vi "Update Accessory Info Tree.vi"(8 "error in":errorcluster, 9 "Devs with Inserted/Removed Accessories":string[](array[string]), 10 "All Devices":tag[](array[tag]), 11 "Accessory Info Tree":refnum<vi>) -> (0 "error out":errorcluster)   [LabVIEW 2022 SP3]
doc: "This VI updates a tree control to display DAQmx device and accessory information."
uses:
  <resource>/objmgr/daqmx.rc
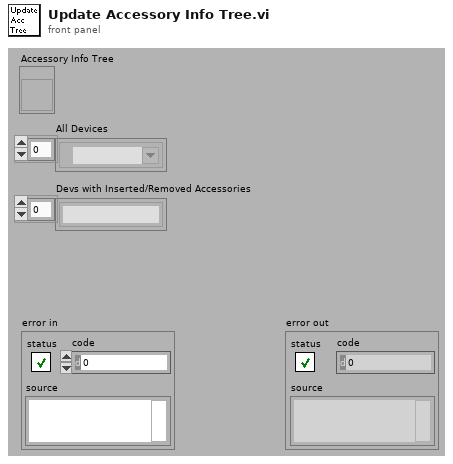
[diagram p1: front panel]
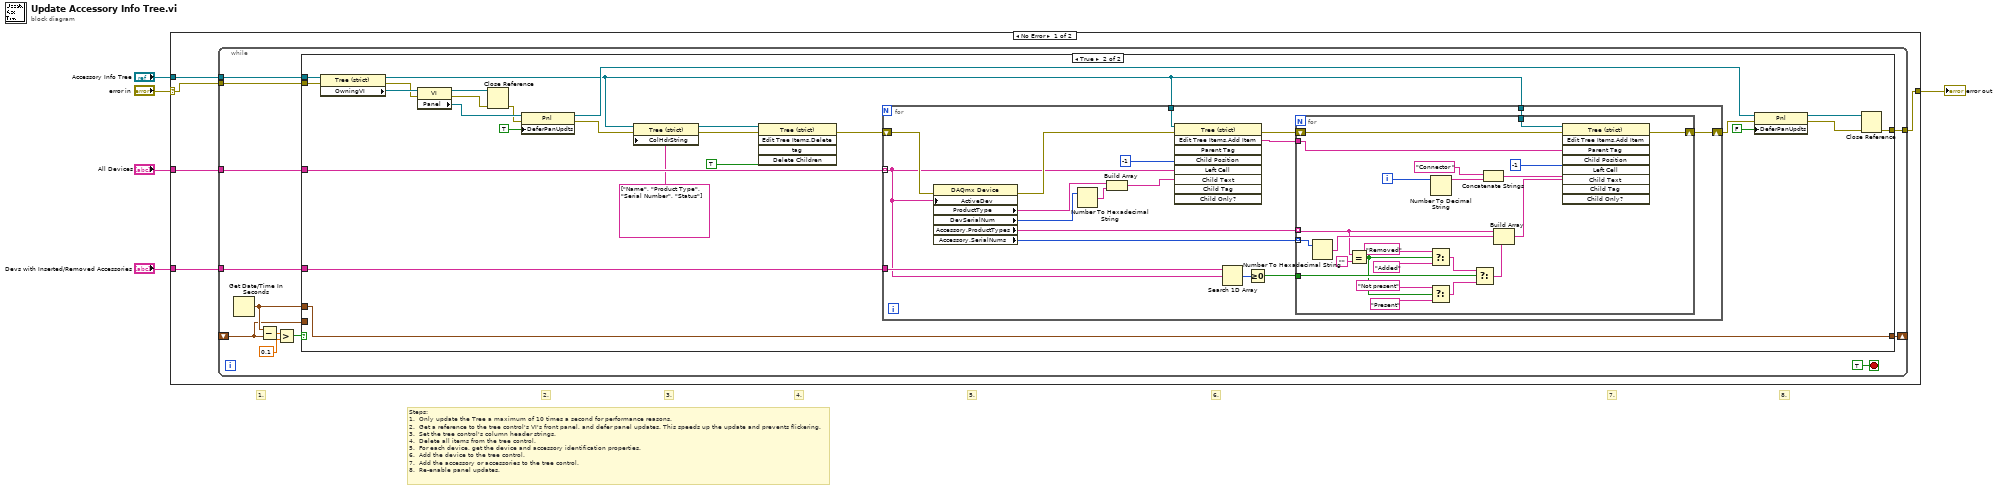
[diagram p0: block diagram]
diagram:
  # "1."
  # "8."
  # "7."
  # "6."
  # "5."
  # "4."
  # "3."
  # "Steps:\n1.  Only update the Tree a maximum of 10 times a second for performance reasons.\n2.  Get a reference to the tree control's VI's front panel, and defer panel updates. This speeds up the update and prevents flickering.\n3.  Set the tree control's column header strings.\n4.  Delete all items from the tree control.\n5.  For each device, get the device and accessory identification properties.\n6.  Add the device to the tree control.\n7.  Add the accessory or accessories to the tree control.\n8.  Re-enable panel updates."
  # "2."
  n1 = case shown="No Error" "error in" {
    selector: "error in" -> [w10 w91]
    tunnel: "Accessory Info Tree" -> [w9 _]
    tunnel: "All Devices" -> [w7 _]
    tunnel: [w8 w91] -> w2
    tunnel: "Devs with Inserted/Removed Accessories" -> [w6 _]
    frame No Error {
      n2 = while {
        tunnel: w10 -> [w22]
        tunnel: w9 -> [w21]
        tunnel: [w20] -> w8
        tunnel: w7 -> [w19]
        tunnel: w6 -> [w18]
        shift-right: [w13] -> _
        shift-left: _ -> [w12]
        stop <- TRUE stop-if-true
        n3 = Get Date/Time In Seconds() -> (seconds since 1Jan1904=w14:timestamp)
        n4 = Subtract(x=w14, y=w12) -> (x-y=w16:dbl)
        n5 = Greater?(x=w16, y=0.1) -> (0:w11:bool)
        n6 = case shown="True" w11 {
          tunnel: w22 -> [w24 w49]
          tunnel: w21 -> [_ w42]
          tunnel: [w24 w33] -> w20
          tunnel: w19 -> [_ w32]
          tunnel: w18 -> [_ w31]
          tunnel: w14 -> [_ w25]
          tunnel: [w23 w25] -> w13
          tunnel: w12 -> [w23 _]
          frame False {
          }
          frame True {
            n7 = property class="Tree (strict)"(reference=w42, error in=w49) -> (reference out=w26:refnum<vi>, error out=w44:errorcluster, "OwningVI"=w47:refnum<vi>)
            n8 = property class="VI"(reference=w47, error in=w44) -> (reference out=w43:refnum<vi>, error out=w41:errorcluster, "Panel"=w46:refnum<vi>)
            n9 = Close Reference(reference=w43, error in (no error)=w41) -> (error out=w40:errorcluster)
            n10 = property class="Pnl"(reference=w46, error in=w40, "DeferPanUpdts"=TRUE ("Defer Panel Updates")) -> (reference out=w36:refnum<vi>, error out=w30:errorcluster)
            n11 = property class="Tree (strict)"(reference=w26, error in=w30, "ColHdrString"=string[] ["Name", "Product Type", "Serial Number", "Status"]) -> (reference out=w28:refnum<vi>, error out=w29:errorcluster)
            n12 = invoke class="Tree (strict)" method="Edit Tree Items.Delete"(reference=w28, error in=w29, "Delete Children"=TRUE ("Delete Children?")) -> (error out=w39:errorcluster)  [unwired: 2 in, 4 out]
            n13 = for {
              tunnel: w32 -> [w54] mode=indexing
              shift-right: [w56] -> w37
              shift-left: w39 -> [w67]
              tunnel: w31 -> [w55]
              tunnel: w26 -> [w51]
              tunnel: w26 -> [w50]
              n14 = property class="DAQmx Device"(error in=w67, "ActiveDev"=w54) -> (error out=w66:errorcluster, "ProductType"=w62:string, "DevSerialNum"=w64:u32, "Accessory.ProductTypes"=w60:string[], "Accessory.SerialNums"=w59:u32[])  [unwired: 1 in, 1 out]
              n15 = Number To Hexadecimal String(2:w64) -> (0:w63:string)  [unwired: 1 in]
              n16 = Build Array(w62, w63) -> (w61:string[])
              n17 = invoke class="Tree (strict)" method="Edit Tree Items.Add Item"(reference=w51, error in=w66, "Child Position"=-1, "Left Cell"=w54, "Child Text"=w61) -> (error out=w57:errorcluster, "Edit Tree Items:Add Item"=w58:string)  [unwired: 4 in, 7 out]
              n18 = Search 1D Array(1D array=w55, element=w54) -> (index of element=w53:i32)  [unwired: 1 in]
              n19 = Greater Or Equal To 0?(x=w53) -> (x >= 0?=w52:bool)
              n20 = for {
                tunnel: w60 -> [w78] mode=indexing
                tunnel: w59 -> [w90] mode=indexing
                tunnel: w58 -> [w82]
                shift-right: [w80] -> w56
                shift-left: w57 -> [w81]
                tunnel: w52 -> [w74]
                tunnel: w50 -> [w72]
                i -> [w89]
                n21 = Number To Hexadecimal String(2:w90) -> (0:w86:string)  [unwired: 1 in]
                n22 = Equal?(x=w78, y="" ("Empty String Constant")) -> (x = y?=w68:bool)
                n23 = Select(t="Removed", s=w68, f="Added") -> (s? t:f=w75:string)
                n24 = Select(t="Not present", s=w68, f="Present") -> (s? t:f=w71:string)
                n25 = Number To Decimal String(number=w89) -> (decimal integer string=w87:string)  [unwired: 1 in]
                n26 = Select(t=w75, s=w74, f=w71) -> (s? t:f=w73:string)
                n27 = Concatenate Strings("Connector ", w87) -> (w84:string)
                n28 = Build Array(w78, w86, w73) -> (w83:string[])
                n29 = invoke class="Tree (strict)" method="Edit Tree Items.Add Item"(reference=w72, error in=w81, "Parent Tag"=w82, "Child Position"=-1, "Left Cell"=w84, "Child Text"=w83) -> (error out=w80:errorcluster)  [unwired: 3 in, 8 out]
              }
            }
            n30 = property class="Pnl"(reference=w36, error in=w37, "DeferPanUpdts"=FALSE ("Defer Panel Updates")) -> (reference out=w35:refnum<vi>, error out=w34:errorcluster)
            n31 = Close Reference(reference=w35, error in (no error)=w34) -> (error out=w33:errorcluster)
          }
        }
      }
    }
    frame Error {
    }
  }
  "error out" <- w2
